vi "PID (DBL) 2.vi"(6 "reinitialize? (F)":bool, 7 "output range":cluster{"output high":dbl, "output low":dbl}={"output high"=100.0, "output low"=-100.0} {"output low" format="%.2f"; "output high" format="%.2f"}, 8 "dt (s)":dbl=-1.0 format="%.3f", 9 "PID gains":T1={"proportional gain (Kc)"=1.0, "integral time (Ti, min)"=0.01, "derivative time (Td, min)"=0.0} {"derivative time (Td, min)" format="%.3f"; "integral time (Ti, min)" format="%.3f"; "proportional gain (Kc)" format="%.3f"}, 10 "process variable":dbl format="%.2f", 11 "setpoint":dbl format="%.2f") -> (0 "dt out (s)":dbl format="%.3f", 3 "output":dbl format="%.2f")   [LabVIEW 2009]
doc: "PID algorithm for simple PID applications or high speed control applications that require an efficient algorithm. The PID algorithm features control output range limiting with integrator anti-windup and bumpless controller output for PID gain changes. You can use this polymorphic VI to operate on a single input value or on an array of input values. The DBL instance can be used to implement a single control loop, whereas the DBL Array instance can be used to implement parallel multi-loop control."
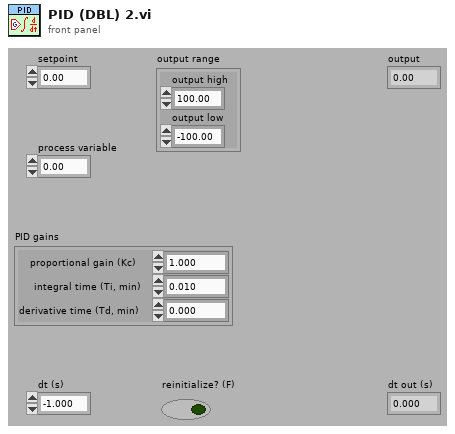
[diagram p1: front panel]
types:
  T1 = cluster{"proportional gain (Kc)":dbl, "integral time (Ti, min)":dbl, "derivative time (Td, min)":dbl}
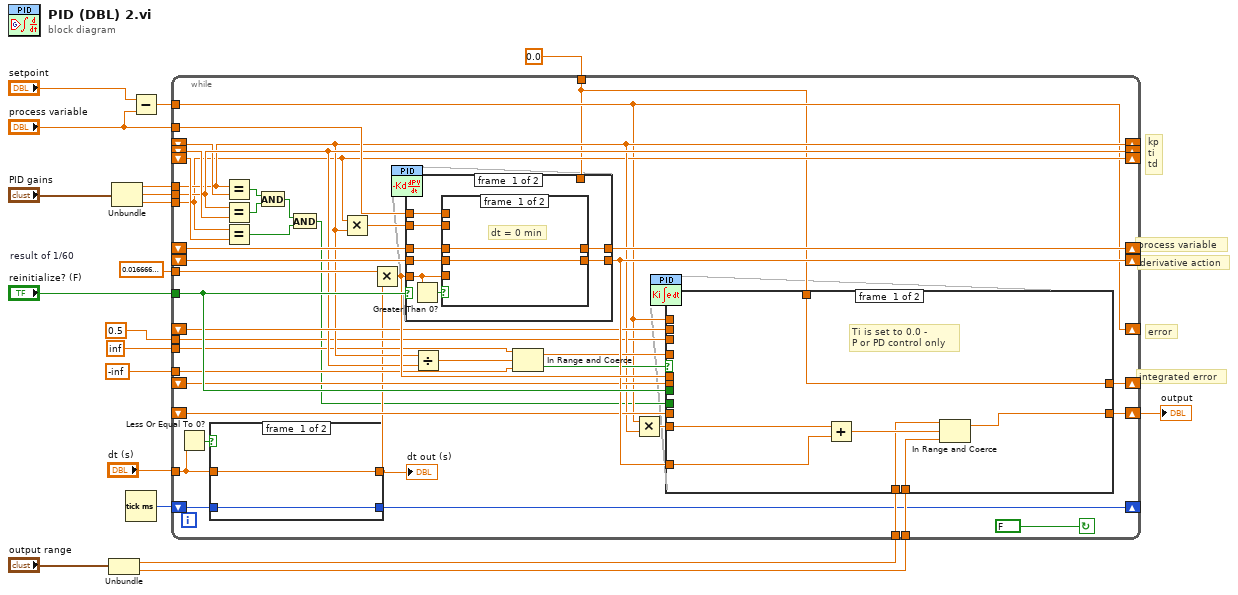
[diagram p0: block diagram]
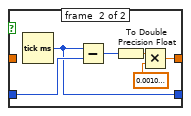
[diagram p2: hidden frame]
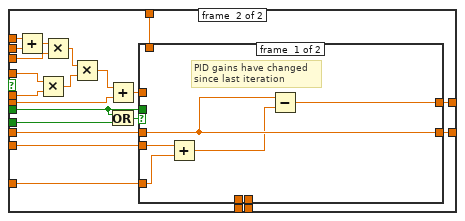
[diagram p3: hidden frame]
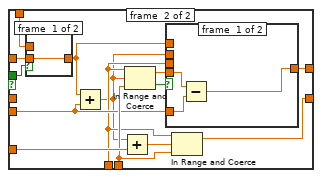
[diagram p4: hidden frame]
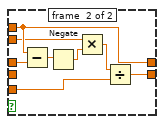
[diagram p7: hidden frame]
diagram:
  w14 = 0.016666666666666666  # result of 1/60
  # "derivative action"
  # "process variable"
  # "kp\nti\ntd"
  # "error"
  # "integrated error"
  n1 = Unbundle("output range") -> ("output high"=w16:dbl, "output low"=w15:dbl)
  n2 = Unbundle("PID gains") -> ("proportional gain (Kc)"=w19:dbl, "integral time (Ti, min)"=w18:dbl, "derivative time (Td, min)"=w17:dbl)
  n3 = Tick Count (ms)() -> (millisecond timer value=w2:u32)
  n4 = Subtract(x="setpoint", y="process variable") -> (x-y=w4:dbl)
  n5 = while {
    tunnel: "reinitialize? (F)" -> [w61]
    shift-left: w2 -> [w27]
    shift-right: [w28] -> _
    shift-right: [w37] -> _
    shift-left: _ -> [w38]
    shift-right: [w39] -> _
    shift-left: _ -> [w58]
    shift-right: [w32] -> _
    shift-left: _ -> [w59]
    tunnel: w19 -> [w37]
    tunnel: w18 -> [w39]
    tunnel: w17 -> [w32]
    tunnel: "dt (s)" -> [w26]
    tunnel: w16 -> [w57]
    tunnel: w15 -> [w56]
    tunnel: "process variable" -> [w55]
    shift-right: [w54] -> _
    shift-left: _ -> [w53]
    shift-right: [w52] -> _
    shift-left: _ -> [w44]
    shift-right: [w51] -> w8
    shift-left: _ -> [w50]
    shift-right: [w31] -> _
    shift-left: _ -> [w49]
    shift-right: [w48] -> _
    shift-left: _ -> [w47]
    tunnel: w14 -> [w41]
    tunnel: 0.5 ("y") -> [w36]
    tunnel: inf ("upper limit") -> [w34]
    tunnel: -inf ("lower limit") -> [w35]
    tunnel: w4 -> [w31]
    tunnel: 0.0 -> [w30]
    stop <- FALSE continue-if-true
    n6 = Less Or Equal To 0?(x=w26) -> (x <= 0?=w25:bool)
    n7 = case shown="True" w25 {
      tunnel: [w63 w66] -> w29
      tunnel: w27 -> [w62 w65]
      tunnel: [w62 w64] -> w28
      tunnel: w26 -> [w63 _]
      frame #0 {
      }
      frame #1 {
        n8 = Tick Count (ms)() -> (millisecond timer value=w64:u32)
        n9 = Subtract(x=w64, y=w65) -> (x-y=w68:u32)
        n10 = To Double Precision Float(number=w68) -> (double precision float=w67:dbl)
        n11 = Multiply(x=w67, y=0.0010000000474974513) -> (x*y=w66:dbl)
      }
    }
    "dt out (s)" <- w29
    n12 = Equal?(x=w37, y=w38) -> (x = y?=w24:bool)
    n13 = Equal?(x=w39, y=w58) -> (x = y?=w23:bool)
    n14 = Equal?(x=w32, y=w59) -> (x = y?=w21:bool)
    n15 = And(x=w24, y=w23) -> (x .and. y?=w22:bool)
    n16 = And(x=w22, y=w21) -> (x .and. y?=w20:bool)
    n17 = Multiply(x=w32, y=w37) -> (x*y=w43:dbl)
    n18 = Multiply(x=w41, y=w29) -> (x*y=w60:dbl)
    n19 = case shown="False" w61 {
      tunnel: w53 -> [w131 _]
      tunnel: w43 -> [w128 _]
      tunnel: w55 -> [w130 w143]
      tunnel: [w127 w143] -> w54
      tunnel: [w129 w142] -> w52
      tunnel: w44 -> [w125 _]
      tunnel: w60 -> [w124 _]
      tunnel: w30 -> [_ w142]
      frame #0 {
        n20 = Greater Than 0?(x=w124) -> (x > 0?=w126:bool)
        n21 = case shown="True" w126 {
          tunnel: w131 -> [w133 w139]
          tunnel: w124 -> [_ w138]
          tunnel: w130 -> [_ w136]
          tunnel: [w132 w137] -> w129
          tunnel: w128 -> [_ w134]
          tunnel: [w133 w136] -> w127
          tunnel: w125 -> [w132 _]
          frame #0 {
            # "dt = 0 min"
          }
          frame #1 {
            n22 = Subtract(x=w136, y=w139) -> (x-y=w141:dbl)
            n23 = Negate(x=w141) -> (-x=w135:dbl)
            n24 = Multiply(x=w134, y=w135) -> (x*y=w140:dbl)
            n25 = Divide(x=w140, y=w138) -> (x/y=w137:dbl)
          }
        }
      }
      frame #1 {
      }
    }
    n26 = Divide(x=w37, y=w39) -> (x/y=w42:dbl)
    n27 = In Range and Coerce(upper limit=w34, x=w42, lower limit=w35) -> (coerced(x)=w46:dbl, In Range?=w45:bool)
    n28 = Multiply(x=w31, y=w37) -> (x*y=w40:dbl)
    n29 = case shown="False" w45 {
      tunnel: w31 -> [_ w97]
      tunnel: w49 -> [_ w98]
      tunnel: w47 -> [_ w95]
      tunnel: [w70 w90] -> w48
      tunnel: w46 -> [_ w81]
      tunnel: w40 -> [w75 w93]
      tunnel: [w76 w89] -> w51
      tunnel: w50 -> [_ w91]
      tunnel: w52 -> [w74 w88]
      tunnel: w61 -> [_ w87]
      tunnel: w20 -> [_ w86]
      tunnel: w60 -> [_ w80]
      tunnel: w57 -> [w72 w84]
      tunnel: w56 -> [w71 w85]
      tunnel: w36 -> [_ w83]
      tunnel: w30 -> [w70 w82]
      frame #0 {
        # "Ti is set to 0.0 -\nP or PD control only"
        n30 = Add(x=w75, y=w74) -> (x+y=w73:dbl)
        n31 = In Range and Coerce(upper limit=w72, x=w73, lower limit=w71) -> (coerced(x)=w76:dbl)  [unwired: 1 out]
      }
      frame #1 {
        n32 = Add(x=w97, y=w98) -> (x+y=w96:dbl)
        n33 = Multiply(x=w81, y=w80) -> (x*y=w79:dbl)
        n34 = Multiply(x=w96, y=w83) -> (x*y=w78:dbl)
        n35 = Multiply(x=w78, y=w79) -> (x*y=w77:dbl)
        n36 = Add(x=w77, y=w95) -> (x+y=w94:dbl)
        n37 = Or(x=w87, y=w86) -> (x .or. y?=w92:bool)
        n38 = case shown="True" w92 {
          tunnel: w94 -> [_ w111]
          tunnel: w93 -> [w101 w106]
          tunnel: w91 -> [w103 _]
          tunnel: w87 -> [_ w113]
          tunnel: [w102 w108] -> w90
          tunnel: [w103 w116] -> w89
          tunnel: w88 -> [w100 w115]
          tunnel: w85 -> [_ w114]
          tunnel: w84 -> [_ w105]
          tunnel: w82 -> [_ w112]
          frame #0 {
            # "PID gains have changed\nsince last iteration"
            n39 = Add(x=w101, y=w100) -> (x+y=w99:dbl)
            n40 = Subtract(x=w103, y=w99) -> (x-y=w102:dbl)
          }
          frame #1 {
            n41 = case shown="True" w113 {
              tunnel: w112 -> [_ w123]
              tunnel: [w122 w123] -> w110
              tunnel: w111 -> [w122 _]
              frame #0 {
              }
              frame #1 {
              }
            }
            n42 = Add(x=w110, y=w106) -> (x+y=w104:dbl)
            n43 = Add(x=w104, y=w115) -> (x+y=w117:dbl)
            n44 = In Range and Coerce(upper limit=w105, x=w104, lower limit=w114) -> (coerced(x)=w107:dbl, In Range?=w109:bool)
            n45 = case shown="False" w109 {
              tunnel: w110 -> [_ w121]
              tunnel: [w118 w121] -> w108
              tunnel: w107 -> [w120 _]
              tunnel: w106 -> [w119 _]
              tunnel: w105 -> [_ _]
              tunnel: w104 -> [_ _]
              frame #0 {
                n46 = Subtract(x=w120, y=w119) -> (x-y=w118:dbl)
              }
              frame #1 {
              }
            }
            n47 = In Range and Coerce(upper limit=w105, x=w117, lower limit=w114) -> (coerced(x)=w116:dbl)  [unwired: 1 out]
          }
        }
      }
    }
  }
  "output" <- w8
